vi "mupExpr sglExpr multiVar example.vi"() -> ()   [LabVIEW 2015]
uses:
  mupExpr/mupExpr.lvclass/mupExpr.ctl
  mupExpr/Eval_MultiVar_SglRes.vi
  mupLib/mupEval.vi
  mupExpr/SetVarVal.vi
  mupLib/mupCheckError.vi
  mupLib/mupLibPath.vi
  mupLib/mupSetVarValue.vi
  <vilib>/Utility/error.llb/Error Cluster From Error Code.vi
  mupExpr/mupExpr.lvclass
panel:
  out "error out":errorcluster
  out "Result":dbl format="%#_13g"
  out "Variable Names":string[](array[string])
  in  "Expression":string="sin(w*t+c)"
  in  "Variable Values":dbl[](array[numeric])=[0.0, 1.0, 3.141592654] format="%#_13g"
  # "This example demonstrates the evaluation of a multi-variable expression.\n\n- Enter an expression composed of any number of variables\n- Enter the value of each variable (variables are listed in alphabetical order)\n- Hit run to evaluate the expression"
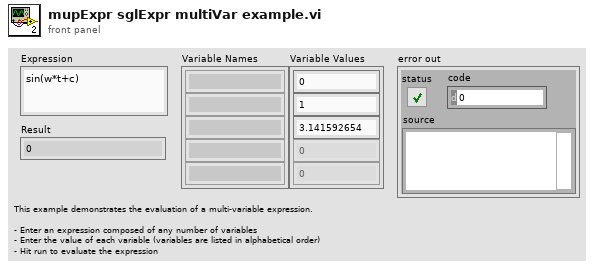
[diagram p1: front panel]
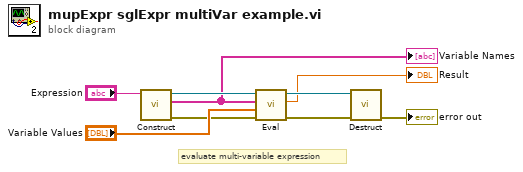
[diagram p0: block diagram]
diagram:
  # "evaluate multi-variable expression"
  n1 = call "Construct.vi"("Expression"="Expression") -> ("error out"=w3:errorcluster, "Variable Names"=w5:string[], "mupExpr out"=w7:refnum<data-value>)  [unwired: 8 in]
  "Variable Names" <- w5
  n2 = call-poly "Eval.vi"("error in (no error)"=w3, "varValues"="Variable Values", "varNames"=w5, "mupExpr in"=w7) -> ("error out"=w2:errorcluster, "Result"=→"Result":dbl, "mupExpr out"=w6:refnum<data-value>)  [unwired: 5 in]
  n3 = call "Destruct.vi"("error in (no error)"=w2, "mupExpr in"=w6) -> ("error out"=→"error out":errorcluster)  [unwired: 9 in]
